vi "FPGA Video Recording (Host).vi"() -> ()   [LabVIEW 2013]
doc: "This is the host VI for the 10-Tap 8-Bit Camera with DRAM example. This example demonstrates how to acquire images from a 10-tap, 8-bit, extended configuration, Camera Link camera and display the images on the host. This example supports area scan and line scan cameras for both continuous and finite acquisitions.\n\nThis example also demonstrates the use of DRAM as a frame buffer for very high speed acquisitions. Data packing and flow-control are also employed to maximize use of the available DRAM and FIFOs in terms of both memory space and performance.\n\nAdditionally, the example demonstrates the serial server, which allows third-party camera configuration utilities to communicate with the camera using the Camera Link serial interface while this VI is running."
uses:
  <vilib>/userdefined/High Color/nirio_resource_hc.ctl
  <vilib>/rvi/interface/common/niFpgaWaitOnOcc.vi
  <vilib>/FPGAPlugInAG/PCIe-1473R/niLvFpga_Open_PCIe-1473R.vi
  <vilib>/rvi/interface/common/dynamic/niFpgaDynamicAddResources.vi
  <vilib>/FPGAPlugInAG/Dynamic/niLvFpga_Reset_Dynamic.vi
  <vilib>/Utility/error.llb/Error Cluster From Error Code.vi
  <vilib>/rvi/errors/niLvFpgaAdjustHostInterfaceError.vi
  <vilib>/FPGAPlugInAG/Dynamic/niLvFpga_Run_Dynamic.vi
  <vilib>/FPGAPlugInAG/Dynamic/niLvFpga_Close_Dynamic.vi
  <vilib>/rvi/interface/nirviOpenFPGA/nirviOpenFPGA.xnode
  FPGA Bitfiles/ImageAcquisitionWithDRAM.lvbitx
  <vilib>/rvi/interface/nirviMethod/nirviMethod.xnode
  <vilib>/rvi/interface/nirviReadWriteControl/nirviReadWriteControl.xnode
  <vilib>/rvi/interface/nirviCloseFPGA/nirviCloseFPGA.xnode
  <vilib>/rvi/interface/Simulation/niFpgaSimulationCallBeginRW.vi
  <vilib>/rvi/errors/niLvFpgaMergeErrorWithErrorCode.vi
  NiFpgaLv.dll
  <vilib>/FPGAPlugInAG/Dynamic/niLvFpga_ConfigureFifo_Dynamic.vi
  <vilib>/FPGAPlugInAG/Dynamic/niLvFpga_StartFifo_Dynamic.vi
  <vilib>/FPGAPlugInAG/Dynamic/niLvFpga_ReadFifo_Dynamic.vi
panel:
  out "DMA Full":bool
  out "Codec Chosen":string="Motion JPEG (NI Vision)"
  in  "Codec index":i32=4
  out "Installed Codecs":string[](array[string])=["Microsoft Video 1", "Intel IYUV codec", "Cinepak Codec by Radius", "FF Video Codec 1 (FFV1) (NI Vision)", "Motion JPEG (NI Vision)", "Y800 Uncompressed Grey Scale (NI Vision)", "YUV 4:2:0 Planar (NI Vision)"]
  out "AVI Path":path=path "F:/Live_Data/20130925_saveFPGAframes/20130925_saveFPGAframes_test1/20130925_saveFPGAframes_test5JPEG5fps.avi"
  in  "AVI fps":u32=5
  out "# of lost frames":u32
  in  "Record?":bool
  in  "DMA Buffer Size\n(In Images)":u32=64 caption="DMA Buffer Size"
  in  "Signal Mapping":T1(ring)=enum."Basler 10-tap"
  out "Acq In Progress":bool=TRUE
  in  "Line Scan":bool
  in  "Frames To Acquire":u32 caption="Frames To Acquire\n(0 = infinite)"
  in  "Cancel":bool
  out "Acq'd Frame Width":u32=2040
  in  "Stopped":bool=TRUE
  in  "RIO Device":T2="RIO0"
  out "DMA Write Timeout":bool
  in  "Start Serial Server":bool=TRUE
  out "Frames Acq'd":u32=49
  out "Acq'd Frame Height":u32=1088
  out "Image":T3(plugin-control)
  in  "Acquire":bool
  in  "Stop":bool
  in  "Image Height":u32=1088 max=65535
  in  "Image Width":u32=2040 max=65535 step=40
  out "Initialized":bool
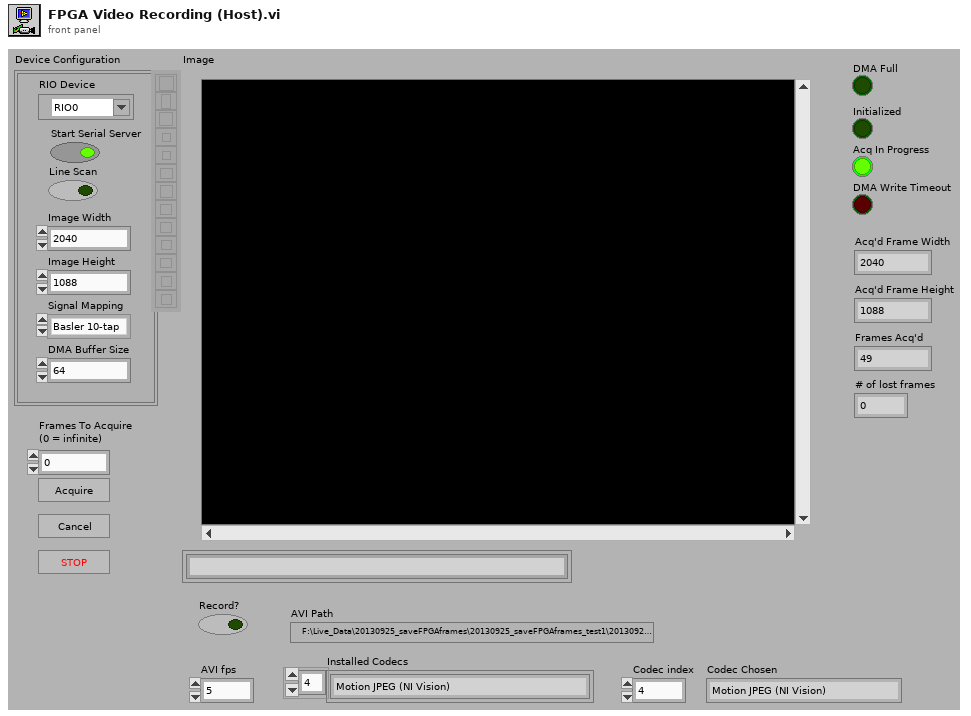
[diagram p1: front panel]
types:
  T1 = enum8{"Standard", "Basler 10-tap", "Vosskühler 10-tap"}
  T2 = typedef "nirio_resource_hc.ctl" = tag
  T3 = typedef "IMAQ Image.ctl" = refnum<image>
  T4 = typedef "Image Type" = u32
  T5 = typedef "IMAQ AVI2 Refnum.ctl" = refnum<k20>
  T6 = enum16{"big-endian, network order", "native, host order", "little-endian"}
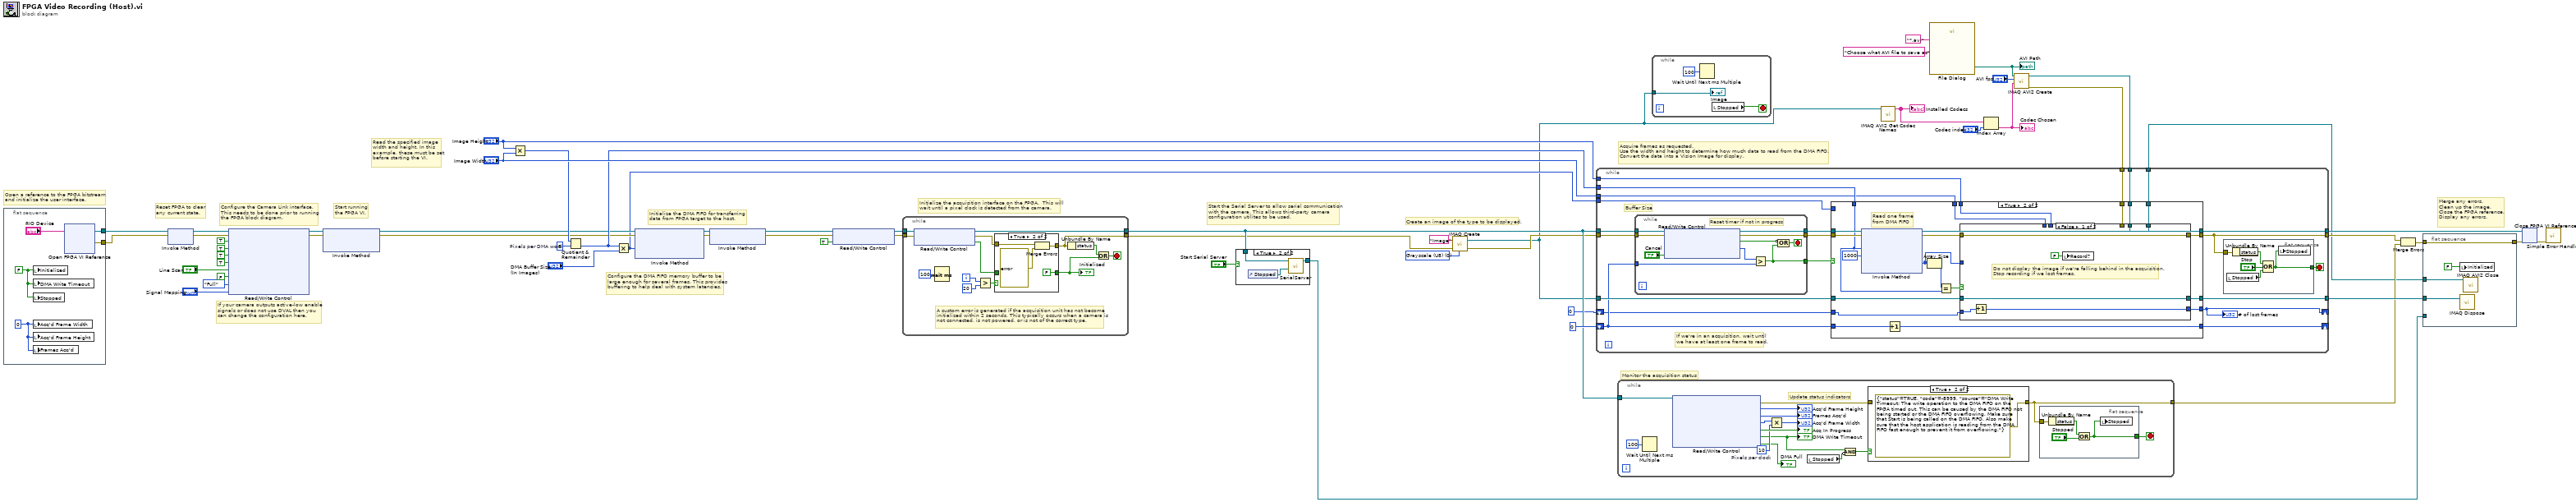
[diagram p0: block diagram]
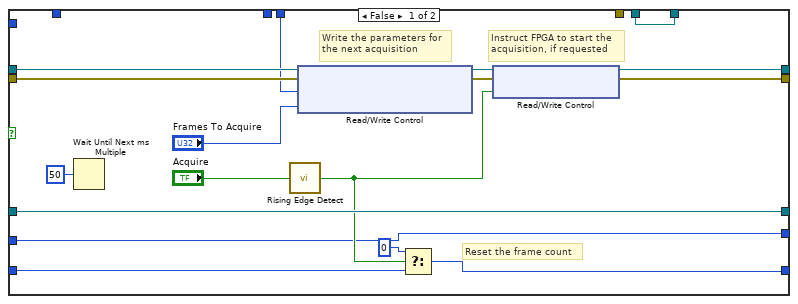
[diagram p4: hidden frame]
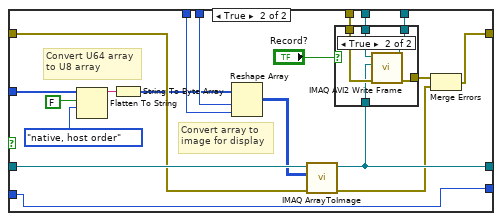
[diagram p5: hidden frame]
diagram:
  w19 = u32 8  # Pixels per DMA word
  w53 = T4 0 items=["Grayscale (U8)", "Grayscale (I16)", "Grayscale (SGL)", "Complex (CSG)", "RGB (U32)", "HSL (U32)", "RGB (U64)", "Grayscale (U16)"] ("Image Type")
  # "If your camera outputs active-low enable\nsignals or does not use DVAL then you \ncan change the configuration here."
  # "Configure the DMA FIFO memory buffer to be\nlarge enough for several frames. This provides\nbuffering to help deal with system latencies."
  # "Start running\nthe FPGA VI."
  # "Reset FPGA to clear\nany current state."
  # "Read the specified image\nwidth and height. In this\nexample, these must be set\nbefore starting the VI."
  # "Merge any errors.\nClean up the image.\nClose the FPGA reference.\nDisplay any errors."
  # "Acquire frames as requested.\nUse the width and height to determine how much data to read from the DMA FIFO.\nConvert the data into a Vision Image for display."
  # "Monitor the acquisition status"
  # "Start the Serial Server to allow serial communication\nwith the camera. This allows third-party camera\nconfiguration utilites to be used."
  # "Create an image of the type to be displayed."
  # "Initialize the acquisition interface on the FPGA.  This will\nwait until a pixel clock is detected from the camera."
  # "Initialize the DMA FIFO for transferring\ndata from FPGA target to the host."
  # "Configure the Camera Link interface.\nThis needs to be done prior to running\nthe FPGA block diagram."
  # "Open a reference to the FPGA bitstream\nand initialize the user interface."
  n1 = flat-sequence {
    tunnel: [w59] -> w44
    tunnel: [w58] -> w57
    frame #0 {
      w62 = u32 0 ("Num Lines Acq'd")
      w61 = FALSE ("stop")
      n2 = local write "Initialized"(w61) -> ()
      n3 = local write "DMA Write Timeout"(w61) -> ()
      n4 = local write "Stopped"(w61) -> ()
      n5 = local write "Acq'd Frame Width"(w62) -> ()
      n6 = local write "Acq'd Frame Height"(w62) -> ()
      n7 = local write "Frames Acq'd"(w62) -> ()
      n8 = xnode "Open FPGA VI Reference"("resource name"="RIO Device") -> ("FPGA VI Reference Out"=w59:refnum<k20>, "error out"=w58:errorcluster)  [unwired: 1 in]
    }
  }
  n9 = xnode "Invoke Method"("FPGA VI Reference In"=w44, "error in"=w57) -> ("FPGA VI Reference Out"=w33:refnum<k20>, "error out"=w36:errorcluster)
  n10 = xnode "Read/Write Control"("FPGA VI Reference In"=w33, "error in"=w36, "CL Config.FVAL Active High"=TRUE ("IO Module Config.CL FVAL Active High"), "CL Config.LVAL Active High"=TRUE ("IO Module Config.CL LVAL Active High"), "CL Config.DVAL Active High"=TRUE ("IO Module Config.CL DVAL Active High"), "CL Config.Spare Active High"=TRUE ("IO Module Config.CL Spare Active High"), "CL Config.Line Scan"="Line Scan", "Acq Control.Ignore DVAL"=FALSE ("CL Config.Line Scan"), "CL Config.Configuration"=enum8{"Base", "Medium", "Full"}."Full", "CL Config.Signal Mapping"="Signal Mapping") -> ("FPGA VI Reference Out"=w37:refnum<k20>, "error out"=w35:errorcluster)
  n11 = xnode "Invoke Method"("FPGA VI Reference In"=w37, "error in"=w35) -> ("FPGA VI Reference Out"=w16:refnum<k20>, "error out"=w15:errorcluster)  [unwired: 1 in]
  n12 = Multiply(x="Image Height", y="Image Width") -> (x*y=w18:u32)
  n13 = Quotient & Remainder(x=w18, y=w19) -> (floor(x/y)=w17:u32)  [unwired: 1 out]
  n14 = Multiply(x=w17, y="DMA Buffer Size\n(In Images)") -> (x*y=w12:u32)
  n15 = xnode "Invoke Method"("FPGA VI Reference In"=w16, "error in"=w15, "Requested Depth"=w12) -> ("FPGA VI Reference Out"=w43:refnum<k20>, "error out"=w42:errorcluster)  [unwired: 1 out]
  n16 = xnode "Invoke Method"("FPGA VI Reference In"=w43, "error in"=w42) -> ("FPGA VI Reference Out"=w28:refnum<k20>, "error out"=w41:errorcluster)
  n17 = xnode "Read/Write Control"("FPGA VI Reference In"=w28, "error in"=w41, "Acq Control.Initialize"=TRUE ("Arm Acquisition")) -> ("FPGA VI Reference Out"=w56:refnum<k20>, "error out"=w55:errorcluster)
  n18 = while {
    tunnel: w56 -> [w70]
    tunnel: w55 -> [w69]
    tunnel: [w68] -> w25
    tunnel: [w72] -> w24
    i -> [w64]
    stop <- w75 stop-if-true
    # "A custom error is generated if the acquisition unit has not become\ninitialized within 2 seconds. This typically occurs when a camera is\nnot connected, is not powered, or is not of the correct type."
    n19 = xnode "Read/Write Control"("FPGA VI Reference In"=w70, "error in"=w69) -> ("FPGA VI Reference Out"=w68:refnum<k20>, "error out"=w67:errorcluster, "Acq Status.Initialized"=w66:bool)
    n20 = Wait (ms)(milliseconds to wait=u32 100) -> ()  [unwired: 1 out]
    n21 = Greater?(x=w64, y=20) -> (0:w65:bool)
    n22 = case shown="True" w65 {
      tunnel: [w77 FALSE] -> w71
      tunnel: w66 -> [w77 _]
      tunnel: w67 -> [w76 w79]
      tunnel: [w76 w81] -> w72
      frame False {
      }
      frame True {
        n23 = Merge Errors(w79, errorcluster {"status"=TRUE, "code"=-8999, "source"="Acquisition Initialization: This error typically occurs when a camera is not properly connected, is not powered, or is not of the correct type."} ("error in")) -> (w81:errorcluster)
      }
    }
    "Initialized" <- w71
    n24 = Unbundle By Name(w72) -> ("status"=w74:bool)
    n25 = Or(x=w74, y=w71) -> (x .or. y?=w75:bool)
  }
  n26 = case shown="True" "Start Serial Server" {
    tunnel: [_ w82] -> w45
    tunnel: w25 -> [_ w83]
    frame False {
    }
    frame True {
      n27 = control-ref of="Stopped"() -> (w84:refnum<vi>)
      n28 = call "SerialServer.vi"("Stop Refnum"=w84, "FPGA VI Reference In"=w83) -> ("FPGA VI Reference Out"=w82:refnum<k20>)  [unwired: 5 in]
    }
  }
  n29 = call "IMAQ Create"("Image Name"="Image", "Image Type"=w53, "error in (no error)"=w24) -> ("New Image"=w4:T3, "error out"=w14:errorcluster)  [unwired: 2 in]
  n30 = while {
    tunnel: w25 -> [w96]
    tunnel: [w99] -> w38
    stop <- w98 stop-if-true
    w89 = u32 10  # Pixels per clock
    # "Update status indicators"
    n31 = Wait Until Next ms Multiple(millisecond multiple=u32 100) -> ()  [unwired: 1 out]
    n32 = xnode "Read/Write Control"("FPGA VI Reference In"=w96) -> ("error out"=w95:errorcluster, "Acq Status.Lines Per Frame"=→"Acq'd Frame Height":u32, "Acq Status.Frames Acq'd"=→"Frames Acq'd":u32, "Acq Status.Clocks Per Line"=w90:u32, "Acq Status.Acq In Progress"=→"Acq In Progress":bool, "Acq Status.DMA Write Timeout"=w87:bool, "DMA Full"=→"DMA Full":bool)  [unwired: 1 in, 1 out]
    "DMA Write Timeout" <- w87
    n33 = Multiply(x=w90, y=w89) -> (x*y=→"Acq'd Frame Width":u32)
    n34 = local read "Stopped"() -> (w86:bool)
    n35 = Compound Arithmetic op=AND(w87, invert w86) -> (w88:bool)
    n36 = case shown="True" w88 {
      tunnel: w95 -> [w104 _]
      tunnel: [w104 errorcluster {"status"=TRUE, "code"=-8999, "source"="DMA Write Timeout: The write operation to the DMA FIFO on the FPGA timed out. This can be caused by the DMA FIFO not being started or the DMA FIFO overflowing. Make sure that Start is being called on the DMA FIFO. Also make sure that the host application is reading from the DMA FIFO fast enough to prevent it from overflowing."} ("error out")] -> w99
      frame False {
      }
      frame True {
      }
    }
    n37 = flat-sequence {
      tunnel: w99 -> [w103]
      tunnel: [w101] -> w98
      frame #0 {
        n38 = Unbundle By Name(w103) -> ("status"=w102:bool)
        n39 = Or(x=w102, y="Stopped") -> (x .or. y?=w101:bool)
        n40 = local write "Stopped"(w101) -> ()
      }
    }
  }
  n41 = while {
    tunnel: w4 -> [w108]
    stop <- w106 stop-if-true
    n42 = Wait Until Next ms Multiple(millisecond multiple=u32 100) -> ()  [unwired: 1 out]
    n43 = local read "Stopped"() -> (w106:bool)
    "Image" <- w108
  }
  n44 = call "IMAQ AVI2 Get Codec Names"("Image"=w4) -> ("Codec Names"=w6:string[])  [unwired: 9 in, 1 out]
  "Installed Codecs" <- w6
  n45 = call "File Dialog"("prompt"="Choose what AVI file to save as", "pattern (all files)"="*.avi" ("pattern label")) -> ("selected path"=w9:path)  [unwired: 10 in, 3 out]
  "AVI Path" <- w9
  n46 = Index Array(array=w6, index="Codec index") -> (element=w10:string)
  "Codec Chosen" <- w10
  n47 = call "IMAQ AVI2 Create"("Codec"=w10, "Frames Per Second"="AVI fps", "AVI Path"=w9) -> ("error out"=w2:errorcluster, "AVI Refnum"=w3:T5)  [unwired: 7 in]
  n48 = while {
    tunnel: w25 -> [w121]
    tunnel: w14 -> [w120]
    tunnel: w17 -> [w129]
    tunnel: "Image Height" -> [w128]
    tunnel: "Image Width" -> [w127]
    tunnel: w4 -> [w126]
    tunnel: [w124] -> w39
    tunnel: [w125] -> w52
    tunnel: [w122] -> w47
    shift-right: [w116] -> _
    shift-left: u32 0 -> [w115]
    shift-right: [w114] -> _
    shift-left: u32 0 -> [w113]
    tunnel: w12 -> [w112]
    tunnel: w3 -> [w111]
    tunnel: w2 -> [w110]
    tunnel: [w109] -> w1
    stop <- w123 stop-if-true
    # "Buffer Size"
    # "If we're in an acquisition, wait until\nwe have at least one frame to read."
    n49 = while {
      tunnel: w121 -> [w136]
      tunnel: w120 -> [w135]
      tunnel: [w133] -> w119
      tunnel: [w134] -> w118
      tunnel: w115 -> [w139]
      tunnel: [w137] -> w117
      stop <- w138 stop-if-true
      # "Reset timer if not in progress"
      n50 = xnode "Read/Write Control"("FPGA VI Reference In"=w136, "error in"=w135, "Acq Control.Cancel Acq"="Cancel") -> ("FPGA VI Reference Out"=w134:refnum<k20>, "error out"=w133:errorcluster, "Acq Status.Acq In Progress"=w130:bool, "Acq Status.Frames Acq'd"=w132:u32)
      n51 = Greater?(x=w132, y=w139) -> (0:w137:bool)
      n52 = Compound Arithmetic op=OR(invert w130, w137) -> (w138:bool)
    }
    n53 = case shown="True" w117 {
      tunnel: w118 -> [w157 w175]
      tunnel: w119 -> [w156 w174]
      tunnel: w129 -> [_ w164]
      tunnel: w128 -> [w150 w182]
      tunnel: w127 -> [_ w181]
      tunnel: w126 -> [w161 w180]
      tunnel: [w152 w178] -> w124
      tunnel: [w155 w177] -> w125
      tunnel: [w161 w176] -> w122
      tunnel: w115 -> [w158 w173]
      tunnel: [w160 w172] -> w116
      tunnel: [w146 w171] -> w114
      tunnel: w113 -> [w146 w170]
      tunnel: w112 -> [_ _]
      tunnel: w111 -> [w145 w169]
      tunnel: w110 -> [_ w168]
      tunnel: [w145 w167] -> w109
      frame False {
        # "Reset the frame count"
        # "Instruct FPGA to start the\nacquisition, if requested"
        # "Write the parameters for\nthe next acquisition"
        n54 = Wait Until Next ms Multiple(millisecond multiple=u32 50) -> ()  [unwired: 1 out]
        n55 = call "Rising Edge Detect.vi"("Input"="Acquire") -> ("Pulse"=w147:bool)  [unwired: 4 in]
        n56 = xnode "Read/Write Control"("FPGA VI Reference In"=w157, "error in"=w156, "Acq Control.Line Scan Height"=w150, "Acq Control.Frames To Acq"="Frames To Acquire") -> ("FPGA VI Reference Out"=w154:refnum<k20>, "error out"=w153:errorcluster)
        n57 = Select(t=u32 0, s=w147, f=w158) -> (s? t:f=w160:u32)
        n58 = xnode "Read/Write Control"("FPGA VI Reference In"=w154, "error in"=w153, "Acq Control.Acquire"=w147) -> ("FPGA VI Reference Out"=w155:refnum<k20>, "error out"=w152:errorcluster)
      }
      frame True {
        # "Read one frame\nfrom DMA FIFO"
        n59 = xnode "Invoke Method"("FPGA VI Reference In"=w175, "error in"=w174, "Number of Elements"=w164, "Timeout (ms)"=1000) -> ("FPGA VI Reference Out"=w177:refnum<k20>, "error out"=w179:errorcluster, "Data"=w162:u64[])  [unwired: 1 out]
        n60 = Increment(x=w173) -> (x+1=w172:u32)
        n61 = Array Size(array=w162) -> (size(s)=w165:i32)
        n62 = Equal?(x=w165, y=w164) -> (x = y?=w163:bool)
        n63 = case shown="False" w163 {
          tunnel: w182 -> [_ w207]
          tunnel: w181 -> [_ w206]
          tunnel: w180 -> [w188 w205]
          tunnel: w179 -> [w187 w204]
          tunnel: [w187 w190] -> w178
          tunnel: [w188 w197] -> w176
          tunnel: w162 -> [_ w201]
          tunnel: [w186 w195] -> w171
          tunnel: w170 -> [w185 w195]
          tunnel: w169 -> [w183 w194]
          tunnel: w168 -> [_ w193]
          tunnel: [w183 w189] -> w167
          frame False {
            # "Do not display the image if we're falling behind in the acquisition.\nStop recording if we lost frames."
            n64 = Increment(x=w185) -> (x+1=w186:u32)
            n65 = local write "Record?"(FALSE ("Record?")) -> ()
          }
          frame True {
            # "Convert U64 array\nto U8 array"
            # "Convert array to\nimage for display"
            n66 = Flatten To String(anything=w201, prepend array or string size? (T)=FALSE, byte order (0:big-endian, network order)=T6."native, host order") -> (data string=w199:string)  [unwired: 1 in, 2 out]
            n67 = String To Byte Array(string=w199) -> (unsigned byte array=w198:u8[])
            n68 = Reshape Array(w198, w207, w206) -> (w203:u8[][])
            n69 = call "IMAQ ArrayToImage"("error in (no error)"=w204, "Image Pixels (U8)"=w203, "Image"=w205) -> ("error out"=w191:errorcluster, "Image Out"=w197:T3)  [unwired: 7 in]
            n70 = case shown="True" "Record?" {
              tunnel: w197 -> [_ w212]
              tunnel: [w209 w211] -> w192
              tunnel: w194 -> [w208 w214]
              tunnel: w193 -> [w209 w213]
              tunnel: [w208 w210] -> w189
              frame False {
              }
              frame True {
                n71 = call "IMAQ AVI2 Write Frame"("error in (no error)"=w213, "Image"=w212, "AVI Refnum"=w214) -> ("error out"=w211:errorcluster, "AVI Refnum (duplicate)"=w210:T5)  [unwired: 6 in, 1 out]
              }
            }
            n72 = Merge Errors(w192, w191) -> (w190:errorcluster)
          }
        }
      }
    }
    "# of lost frames" <- w114
    n73 = flat-sequence {
      tunnel: w124 -> [w142]
      tunnel: [w141] -> w123
      frame #0 {
        n74 = local read "Stopped"() -> (w140:bool)
        n75 = Unbundle By Name(w142) -> ("status"=w143:bool)
        n76 = Compound Arithmetic op=OR(w143, "Stop", w140) -> (w141:bool)
        n77 = local write "Stopped"(w141) -> ()
      }
    }
  }
  n78 = Merge Errors(w39, w38) -> (w40:errorcluster)
  n79 = flat-sequence {
    tunnel: w40 -> [w217]
    tunnel: [w217] -> w49
    tunnel: w47 -> [w218]
    tunnel: w45 -> [_]
    tunnel: w1 -> [w215]
    frame #0 {
      n80 = local write "Initialized"(FALSE ("Module Enabled")) -> ()
      n81 = call "IMAQ Dispose"("Image"=w218) -> ()  [unwired: 5 in, 1 out]
      n82 = call "IMAQ AVI2 Close"("AVI Refnum"=w215) -> ()  [unwired: 10 in, 1 out]
    }
  }
  n83 = xnode "Close FPGA VI Reference"("FPGA VI Reference In"=w52, "error in"=w49) -> ("error out"=w46:errorcluster)
  n84 = call <vilib>:"Simple Error Handler.vi"("error in (no error)"=w46) -> ()  [unwired: 4 in, 5 out]
